vi "MS SQL_InRFID_STN30.vi"(6 "RFID":string, 7 "OP20_HOSE_TEST":T1, 8 "error in (no error)":errorcluster, 11 "Ref in":T2={"MS SQL Connection"=refnum, "UDL File"=path "", "Time"="", "DCODE"="", "WIP+1"=0, "MC No?"=0, "POKAYOKE?"=FALSE, "Expected Result"="", "Result [Status]"="", "Clock"=0.0, "RFID"="", "WIP Queue"=refnum, "TS Parameter"={"ProfitCenterCode"="", "LineCode"="", "WorkOrderNumber"="", "Model"="", "Model_with_Prefix"="", "VendorCode"="", "SetParameterDateCode"="", "PokaYoke"=0, "Target"=1, "Live_DateCode"="", "CustomerPartNumber"="", "Hand"="", "sBarcode"=FALSE, "FCA"=0, "Ent_Stamp"=timestamp(0 s since 1904-01-01), "STS_CD"=0.0}, "Data_Queue"=[], "RFID Serial No."=""} {"TS Parameter"."FCA" format="%01d"; "TS Parameter"."Target" min=1 max=100000; "TS Parameter"."PokaYoke" min=0 max=1}) -> (0 "error out":errorcluster, 1 "Message":picture, 2 "Saved?":bool, 3 "Ref Out":T2={"MS SQL Connection"=refnum, "UDL File"=path "", "Time"="", "DCODE"="", "WIP+1"=0, "MC No?"=0, "POKAYOKE?"=FALSE, "Expected Result"="", "Result [Status]"="", "Clock"=0.0, "RFID"="", "WIP Queue"=refnum, "TS Parameter"={"ProfitCenterCode"="", "LineCode"="", "WorkOrderNumber"="", "Model"="", "Model_with_Prefix"="", "VendorCode"="", "SetParameterDateCode"="", "PokaYoke"=0, "Target"=1, "Live_DateCode"="", "CustomerPartNumber"="", "Hand"="", "sBarcode"=FALSE, "FCA"=0, "Ent_Stamp"=timestamp(0 s since 1904-01-01), "STS_CD"=0.0}, "Data_Queue"=[], "RFID Serial No."=""} {"TS Parameter"."FCA" format="%01d"; "TS Parameter"."Target" min=1 max=100000; "TS Parameter"."PokaYoke" min=0 max=1})   [LabVIEW 2020]
uses:
  Controls/TD SQL.ctl
  <vilib>/addons/database/Connection.llb/Conn ObjectReference.ctl
  Controls/WIP_State.ctl
  Controls/TS_Parameter.ctl
  <vilib>/addons/database/NI_Database_API.lvlib
panel:
  out "Query":string
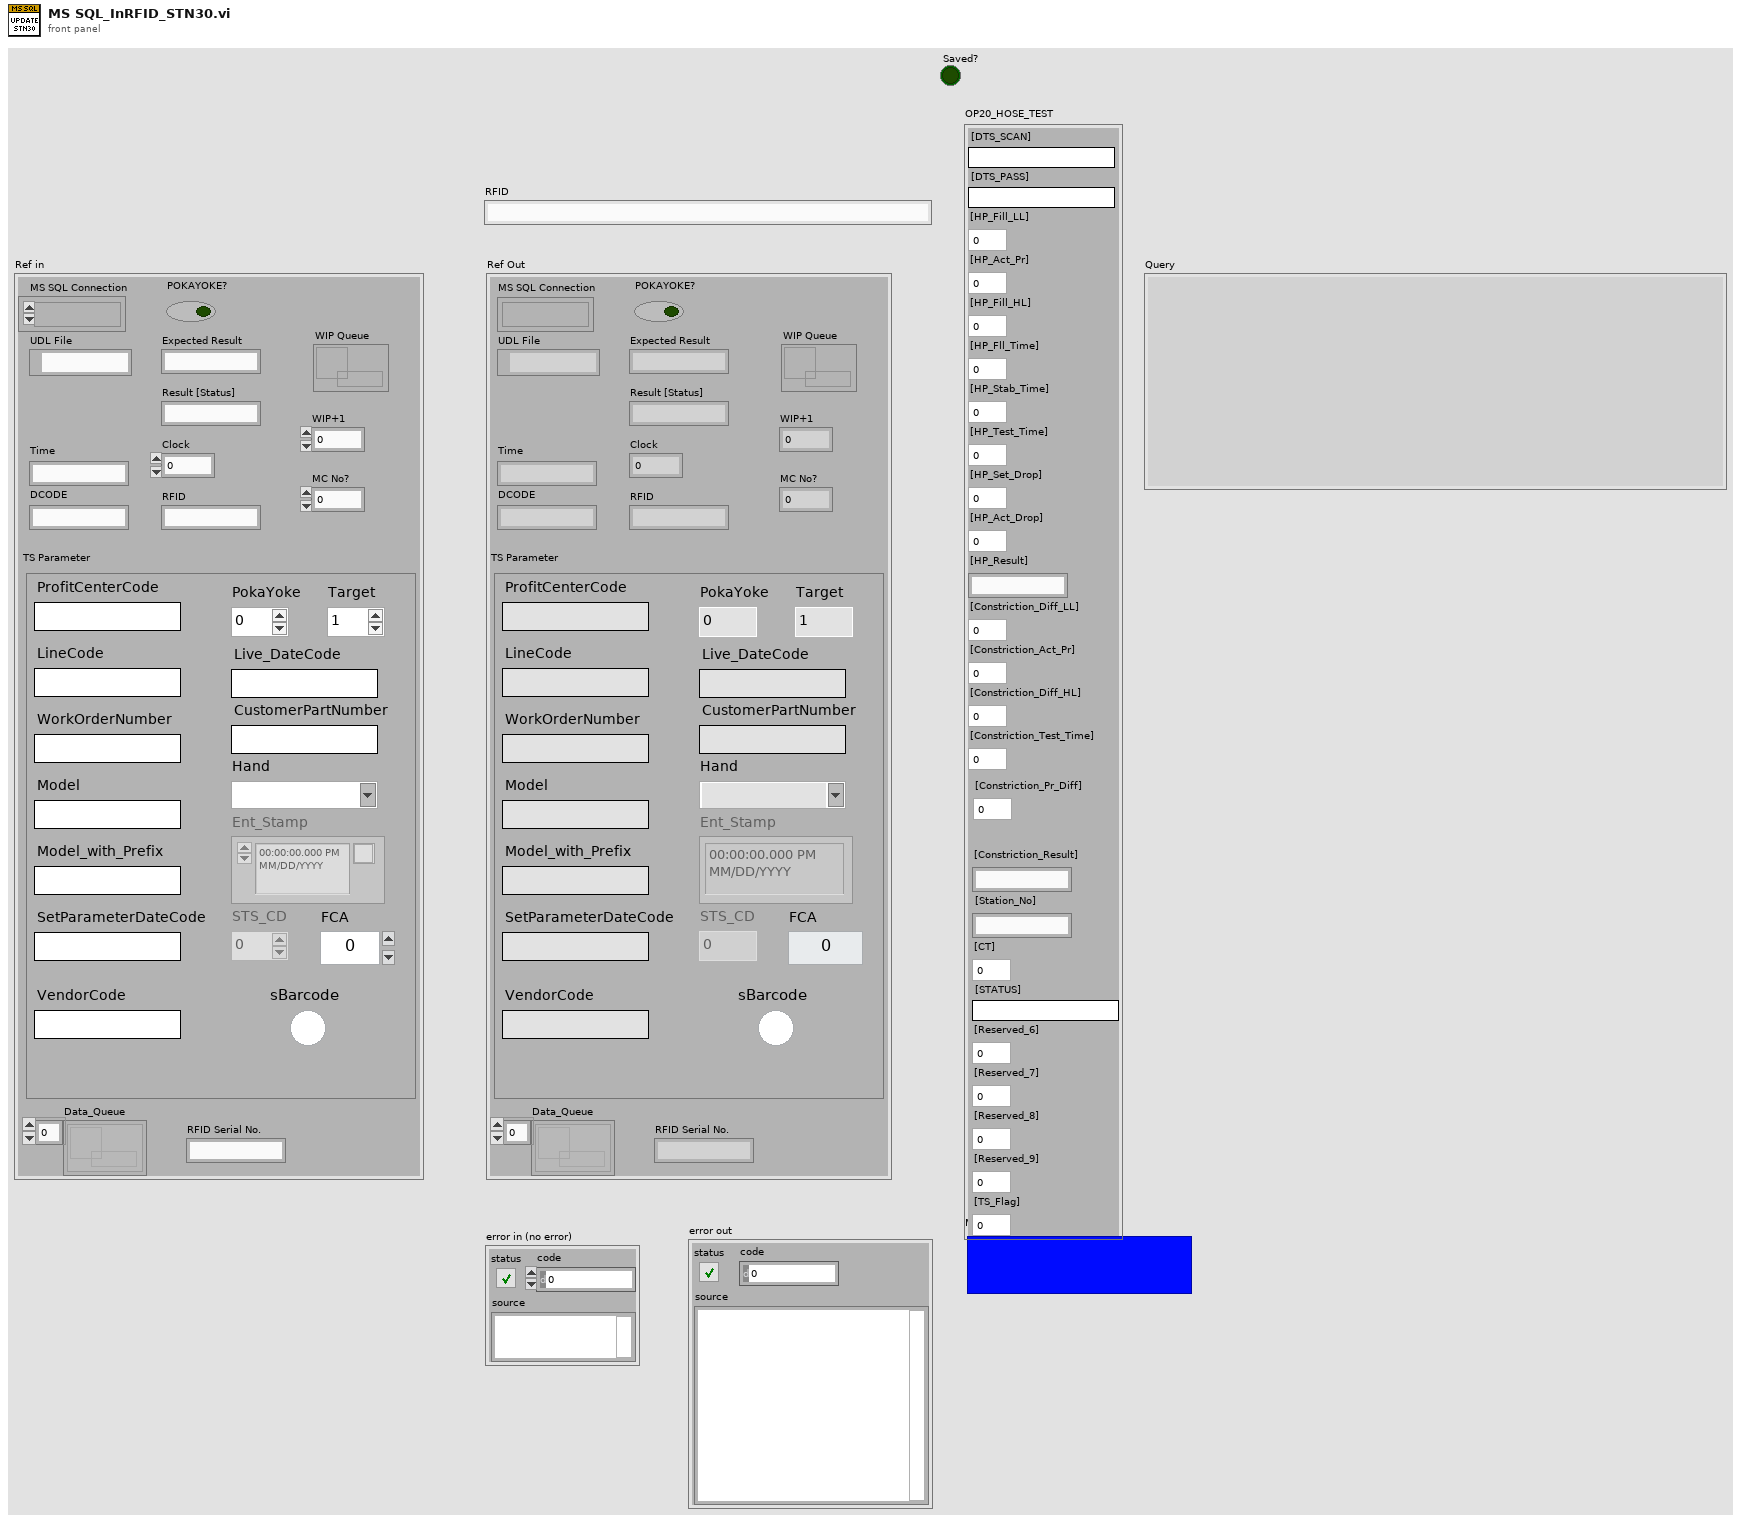
[diagram p1: front panel]
types:
  T1 = cluster{"[DTS_SCAN]":string, "[DTS_PASS]":string, "[HP_Fill_LL]":dbl, "[HP_Act_Pr]":dbl, "[HP_Fill_HL]":dbl, "[HP_Fll_Time]":dbl, "[HP_Stab_Time]":dbl, "[HP_Test_Time]":dbl, "[HP_Set_Drop]":dbl, "[HP_Act_Drop]":dbl, "[HP_Result]":string, "[Constriction_Diff_LL]":dbl, "[Constriction_Act_Pr]":dbl, "[Constriction_Diff_HL]":dbl, "[Constriction_Test_Time]":dbl, "[Constriction_Pr_Diff]":dbl, "[Constriction_Result]":string, "[Station_No]":string, "[CT]":dbl, "[STATUS]":string, "[Reserved_6]":dbl, "[Reserved_7]":dbl, "[Reserved_8]":dbl, "[Reserved_9]":dbl, "[TS_Flag]":dbl}
  T2 = typedef "TD SQL.ctl" = cluster{"MS SQL Connection":T3, "UDL File":path, "Time":string, "DCODE":string, "WIP+1":i64, "MC No?":i32, "POKAYOKE?":bool, "Expected Result":string, "Result [Status]":string, "Clock":dbl, "RFID":string, "WIP Queue":refnum<queue>, "TS Parameter":T4, "Data_Queue":refnum<queue>[], "RFID Serial No.":string}
  T3 = typedef "NI_Database_API.lvlib/Conn ObjectReference.ctl" = refnum<k1>
  T4 = typedef "TS_Parameter.ctl" = cluster{"ProfitCenterCode":string, "LineCode":string, "WorkOrderNumber":string, "Model":string, "Model_with_Prefix":string, "VendorCode":string, "SetParameterDateCode":string, "PokaYoke":i32, "Target":i32, "Live_DateCode":string, "CustomerPartNumber":string, "Hand":string, "sBarcode":bool, "FCA":i32, "Ent_Stamp":timestamp, "STS_CD":dbl}
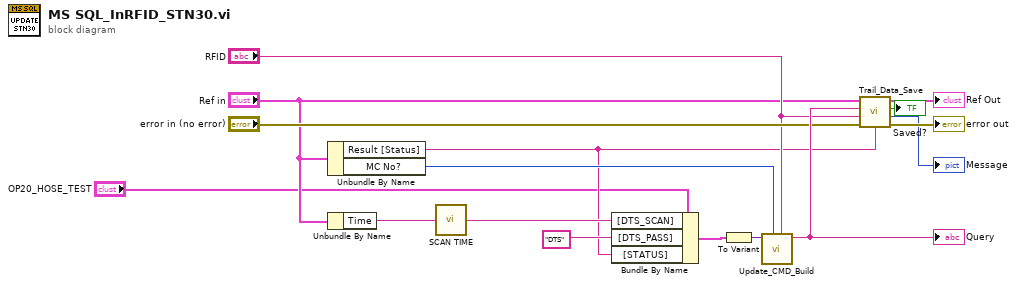
[diagram p0: block diagram]
diagram:
  n1 = Unbundle By Name("Ref in") -> ("Result [Status]"=w3:string, "MC No?"=w5:i32)
  n2 = Unbundle By Name("Ref in") -> ("Time"=w12:string)
  n3 = call "SCAN TIME.vi"("Time in"=w12) -> ("Time out"=w13:string)
  n4 = Bundle By Name(cluster="OP20_HOSE_TEST", "[DTS_SCAN]"=w13, "[DTS_PASS]"="DTS", "[STATUS]"=w3) -> (w15:T1)
  n5 = To Variant(anything=w15) -> (Variant=w16:variant)
  n6 = call "Update_CMD_Build.vi"("RFID"="RFID", "Machine No"=w5, "Variant"=w16) -> ("Update Query"=w11:string)  [unwired: 5 in, 1 out]
  "Query" <- w11
  n7 = call "Trail_Data_Save.vi"("Status"=w3, "error in (no error)"="error in (no error)", "RFID"="RFID", "Query"=w11, "Ref in"="Ref in") -> ("error out"=→"error out":errorcluster, "Message"=→"Message":picture, "Saved?"=→"Saved?":bool, "Ref Out"=→"Ref Out":T2)  [unwired: 1 in]
